vi "Grid_Main_v6.vi"(10 "Final DC":bool, 11 "Settings":T3={"Drift Correction Settings"={"Drift Correction every"=80, "Drift correction Pixels"=256, "Channel index (0-23)"=0, "MaxImagesBack"=2, "Threshold"=2, "Increment"=8, "max applied Drift Correction"=20, "Correct Drift"=TRUE, "Correlate"=0, "Correct z drift"=FALSE, "zdrift \nDuration (s)"=0.0}, "Spectroscopy Setting"={"Imaging Current"=1e-11, "ref Current"=7e-11, "tip Speed (m/s)"=2e-09, "Imaging Bias"=0.02, "ref Bias"=-0.1, "preSTS delay [ms]"=500, "STS z offset"=2e-10, "during Spec Bias (V)"=-0.1, "trigger1 < Hz"=0.0, "trigger 2 >Hz"=0.0, "autoStop"=FALSE, "Spectroscopy"=0, "PLL ON/OFF"=TRUE, "readjust setpoint every "=1, "z Reference (constHeight)"=FALSE, "Lock In"=TRUE}, "Misc"={"File name"="symmetric_node_zOff=200p", "Email when finished"="cornelius.krull@monash.edu,Dhaneesh.Gopalakrishnan@monash.edu,marina.castelli@monash.edu"}, "Grid Settings"={"type"=1, "type order"=1, "X pixel"=0, "Y pixel"=0, "Grid_Parms"={"center X (m)"=0.0, "center Y (m)"=0.0, "width (m)"=0.0, "height (m)"=0.0, "angle (deg)"=0.0}}} {"Grid Settings"."type order" items=["Grid", "Random", "Adam7"]; "Grid Settings"."type" items=["Line", "Grid", "Cloud"]; "Spectroscopy Setting"."Spectroscopy" items=["Bias", "zSpec"]; "Spectroscopy Setting"."trigger 2 >Hz" format="%#_6p"; "Spectroscopy Setting"."trigger1 < Hz" format="%#_6p"; "Spectroscopy Setting"."during Spec Bias (V)" format="%#_5p"; "Spectroscopy Setting"."STS z offset" format="%#_6p"; "Spectroscopy Setting"."ref Bias" format="%#_6p"; "Spectroscopy Setting"."Imaging Bias" format="%#_6p"; "Spectroscopy Setting"."tip Speed (m/s)" format="%.2p"; "Spectroscopy Setting"."ref Current" format="%#_6p"; "Spectroscopy Setting"."Imaging Current" format="%#_6p"; "Drift Correction Settings"."Correlate" items=["first Frame", "successive Frames"]; "Drift Correction Settings"."max applied Drift Correction" min=1 max=100 step=1 format="%.0p"; "Drift Correction Settings"."Threshold" min=1 step=1; "Drift Correction Settings"."Channel index (0-23)" items=["Current"=0, "Z (m)"=14]}) -> (3 "Settings out":T2)   [LabVIEW 2014]
uses:
  <userlib>/Nanonis Prog Interface V5/Nanonis Prog Interface.lvlib
panel:
  in  "resume":T1
  in  "stop":bool
  out "total points":i32
  out "Points taken":i32
  out "ETA":timestamp=timestamp(3575267058.899443 s since 1904-01-01)
  out "remaining time":dbl format="%<%H:%M:%S>t"
  out "Progress":u8(slide)=100 scale=0.0..100.0 scale format="%#.1g"
  out "Last z adjustment":dbl
  out "Last Drift detected (images back)":i32
  out "Y Offset out":sgl format="%#_6p"
  out "X Offset out":sgl format="%#_6p"
  out "Drift Correction Image":picture
  # "RUN smart tilt before starting the GRID\nImg Angle = 0  CHECK CUTOFF\nmove tip to reference point for tip height"
  # "%"
  # "finish the last action and then"
  # "GRID points"
  # "Increase this if no Drift was detected for \na certain number of images"
  # "% of image size"
  # "Only first frame works"
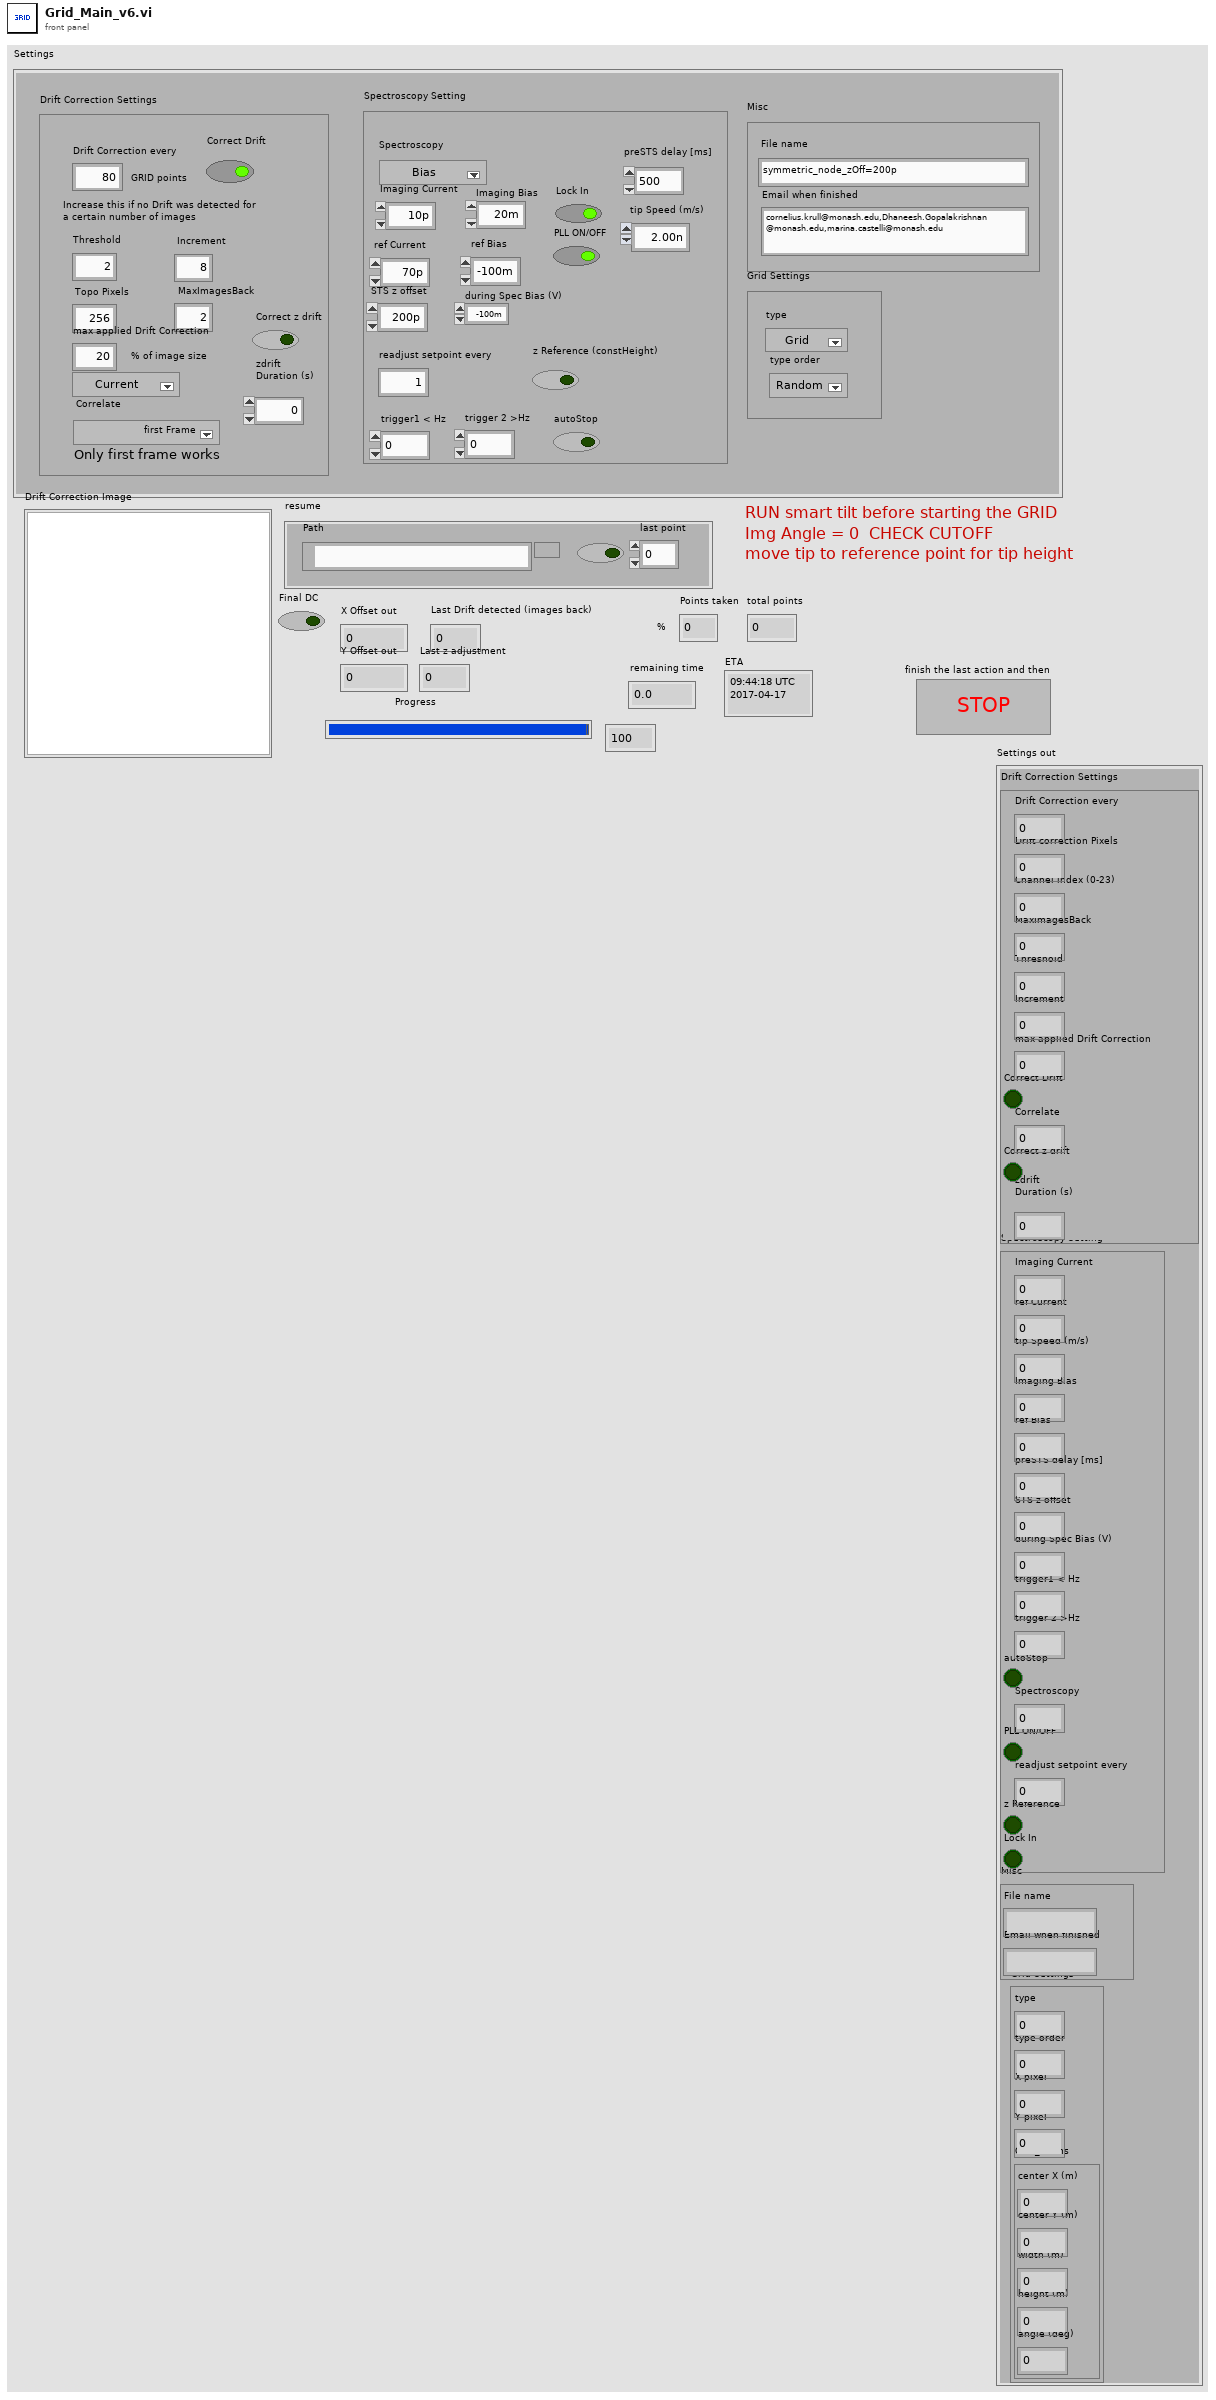
[diagram p1: front panel]
types:
  T1 = cluster{"resume Grid":bool, "Path":path, "last point":i32}
  T2 = cluster{"Drift Correction Settings":cluster{"Drift Correction every":i32, "Drift correction Pixels":i32, "Channel index (0-23)":u8, "MaxImagesBack":i32, "Threshold":i32, "Increment":i32, "max applied Drift Correction":i32, "Correct Drift":bool, "Correlate":u16, "Correct z drift":bool, "zdrift \nDuration (s)":dbl}, "Spectroscopy Setting":cluster{"Imaging Current":dbl, "ref Current":dbl, "tip Speed (m/s)":sgl, "Imaging Bias":dbl, "ref Bias":dbl, "preSTS delay [ms]":u32, "STS z offset":dbl, "during Spec Bias (V)":sgl, "trigger1 < Hz":sgl, "trigger 2 >Hz":sgl, "autoStop":bool, "Spectroscopy":u16, "PLL ON/OFF":bool, "readjust setpoint every ":i32, "z Reference":bool, "Lock In":bool}, "Misc":cluster{"File name":string, "Email when finished":string}, "Grid Settings":cluster{"type":u16, "type order":u16, "X pixel":i32, "Y pixel":i32, "Grid_Parms":cluster{"center X (m)":sgl, "center Y (m)":sgl, "width (m)":sgl, "height (m)":sgl, "angle (deg)":sgl}}}
  T3 = cluster{"Drift Correction Settings":cluster{"Drift Correction every":i32, "Drift correction Pixels":i32, "Channel index (0-23)":u8, "MaxImagesBack":i32, "Threshold":i32, "Increment":i32, "max applied Drift Correction":i32, "Correct Drift":bool, "Correlate":u16, "Correct z drift":bool, "zdrift \nDuration (s)":dbl}, "Spectroscopy Setting":cluster{"Imaging Current":dbl, "ref Current":dbl, "tip Speed (m/s)":sgl, "Imaging Bias":dbl, "ref Bias":dbl, "preSTS delay [ms]":u32, "STS z offset":dbl, "during Spec Bias (V)":sgl, "trigger1 < Hz":sgl, "trigger 2 >Hz":sgl, "autoStop":bool, "Spectroscopy":u16, "PLL ON/OFF":bool, "readjust setpoint every ":i32, "z Reference (constHeight)":bool, "Lock In":bool}, "Misc":cluster{"File name":string, "Email when finished":string}, "Grid Settings":cluster{"type":u16, "type order":u16, "X pixel":i32, "Y pixel":i32, "Grid_Parms":cluster{"center X (m)":sgl, "center Y (m)":sgl, "width (m)":sgl, "height (m)":sgl, "angle (deg)":sgl}}}
  T4 = cluster{"Drift File out":refnum<file>, "zFile":refnum<file>, "BinFile ref":refnum<file>, "xyFile":refnum<file>}
  T5 = cluster{"Drift Correction every":i32, "Drift correction Pixels":i32, "Channel index (0-23)":u8, "MaxImagesBack":i32, "Threshold":i32, "Increment":i32, "max applied Drift Correction":i32, "Correct Drift":bool, "Correlate":u16, "Correct z drift":bool, "zdrift \nDuration (s)":dbl}
  T6 = cluster{"Imaging Current":dbl, "ref Current":dbl, "tip Speed (m/s)":sgl, "Imaging Bias":dbl, "ref Bias":dbl, "preSTS delay [ms]":u32, "STS z offset":dbl, "during Spec Bias (V)":sgl, "trigger1 < Hz":sgl, "trigger 2 >Hz":sgl, "autoStop":bool, "Spectroscopy":u16, "PLL ON/OFF":bool, "readjust setpoint every ":i32, "z Reference":bool, "Lock In":bool}
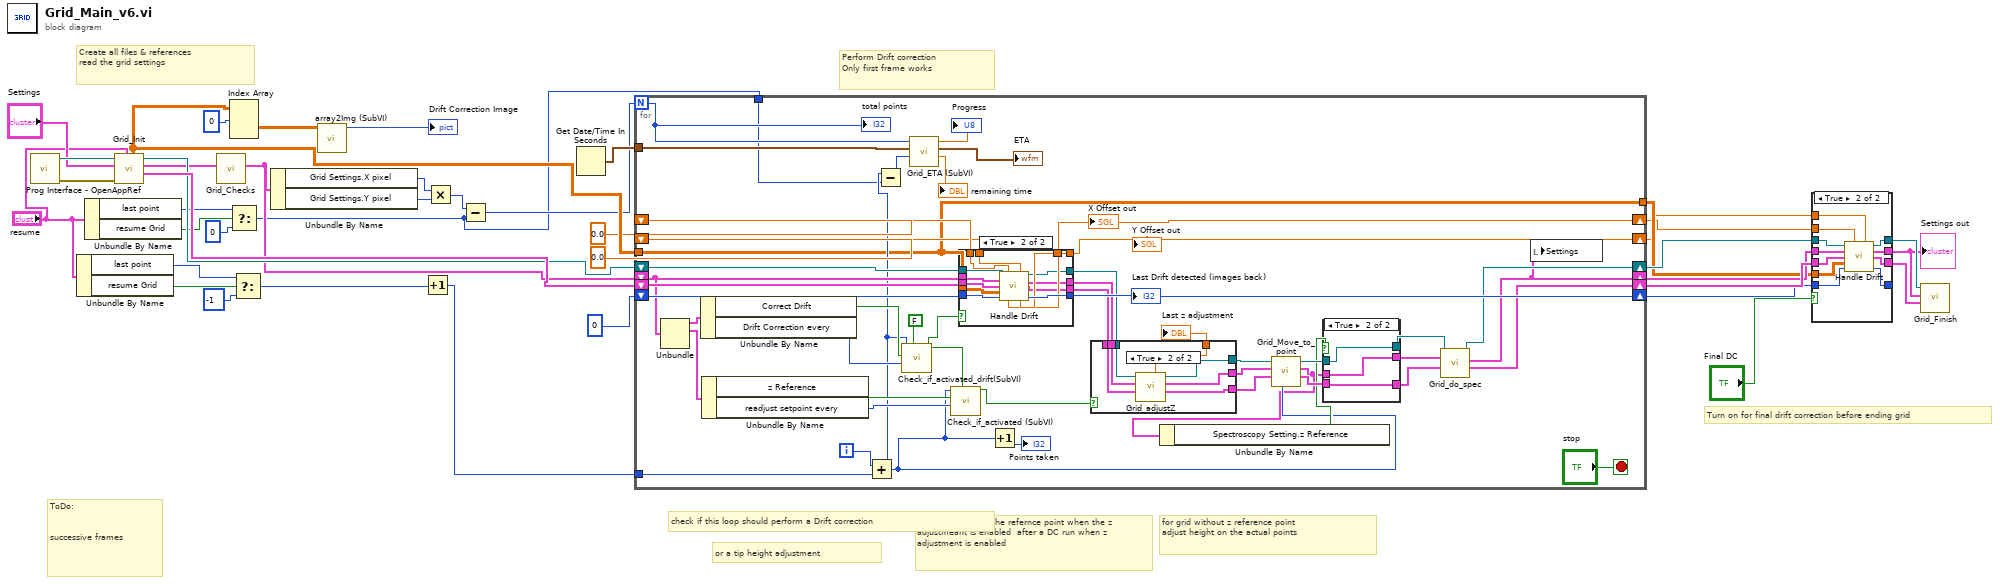
[diagram p0: block diagram]
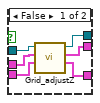
[diagram p3: hidden frame]
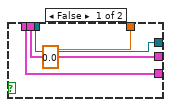
[diagram p4: hidden frame]
diagram:
  # "Turn on for final drift correction before ending grid"
  # "ToDo:\n\n\nsuccessive frames"
  # "Perform Drift correction\nOnly first frame works"
  # "check if this loop should perform a Drift correction"
  # "for grid without z reference point \nadjust height on the actual points"
  # "or a tip height adjustment"
  # "Create all files & references\nread the grid settings"
  # "adjust z height on the refernce point when the z adjustmeant is enabled  after a DC run when z adjustment is enabled"
  n1 = call <userlib>:"Prog Interface - OpenAppRef.vi"() -> ("Error out"=w39:errorcluster, "Application reference"=w40:refnum<vi>)  [unwired: 6 in]
  n2 = Unbundle By Name("resume") -> ("last point"=w21:i32, "resume Grid"=w23:bool)
  n3 = Unbundle By Name("resume") -> ("last point"=w15:i32, "resume Grid"=w17:bool)
  n4 = call "Grid_Init.vi"("resume"="resume", "Error in"=w39, "Settings"="Settings", "Application reference"=w40) -> ("FileRefs"=w37:T4, "Settings out"=w26:T2, "Application ref out"=w36:refnum<vi>, "DC images"=w34:dbl[][][])  [unwired: 3 in, 1 out]
  n5 = call "Grid_Checks.vi"("Settings"=w26) -> ("Settings out"=w25:T2)  [unwired: 10 in]
  n6 = Index Array(array=w34, index (dim 0)=0 ("index (page)")) -> (element=w35:dbl[][])  [unwired: 2 in]
  n7 = Select(t=w15, s=w17, f=0) -> (s? t:f=w12:i32)
  n8 = Select(t=w21, s=w23, f=-1) -> (s? t:f=w20:i32)
  n9 = Unbundle By Name(w25) -> ("Grid Settings.X pixel"=w29:i32, "Grid Settings.Y pixel"=w28:i32)
  n10 = call "array2Img (SubVI).vi"("Rxy"=w35) -> ("new picture"=→"Drift Correction Image":picture)  [unwired: 10 in]
  n11 = Increment(x=w20) -> (x+1=w18:i32)
  n12 = Multiply(x=w29, y=w28) -> (x*y=w13:i32)
  n13 = Subtract(x=w13, y=w12) -> (x-y=w19:i32)
  n14 = Get Date/Time In Seconds() -> (seconds since 1Jan1904=w27:timestamp)
  n15 = for {
    N: w19 -> [w47]
    tunnel: w34 -> [w41]
    shift-right: [w86] -> w7
    shift-left: 0 ("Last Drift out") -> [w85]
    shift-right: [w81] -> w5
    shift-left: sgl 0.0 ("X Offset out") -> [w84]
    shift-right: [w82] -> w4
    shift-left: sgl 0.0 ("Y Offset out") -> [w83]
    tunnel: w27 -> [w72]
    shift-right: [w69] -> w9
    shift-left: w36 -> [w87]
    shift-right: [w43] -> w10
    shift-left: w25 -> [w54]
    shift-right: [w68] -> w11
    shift-left: w37 -> [w88]
    tunnel: w18 -> [w55]
    tunnel: w12 -> [w44]
    tunnel: [w41] -> w6
    i -> [w66]
    stop <- "stop" stop-if-true
    n16 = Unbundle(w54) -> ("Drift Correction Settings"=w53:T5, "Spectroscopy Setting"=w51:T6)  [unwired: 2 out]
    n17 = Unbundle By Name(w53) -> ("Correct Drift"=w52:bool, "Drift Correction every"=w48:i32)
    n18 = Unbundle By Name(w51) -> ("z Reference"=w50:bool, "readjust setpoint every"=w49:i32)
    n19 = Add(x=w66, y=w55) -> (x+y=w45:i32)
    n20 = Subtract(x=w45, y=w44) -> (x-y=w46:i32)
    n21 = call "Check_if_activated_drift(SubVI).vi"("Override"=FALSE, "activate  every  iterations"=w48, "activated?"=w52, "Iteration"=w45) -> ("perform action"=w77:bool)  [unwired: 7 in]
    n22 = call "Grid_ETA (SubVI).vi"("points taken"=w46, "seconds since 1Jan1904"=w72, "points todo"=w47) -> ("Numeric 4"=→"remaining time":dbl, "Time Stamp"=→"ETA":timestamp, "Numeric 3"=→"Progress":dbl)  [unwired: 6 in]
    n23 = call "Check_if_activated (SubVI).vi"("Override"=w77, "activate  every  iterations"=w49, "activated?"=w50, "Iteration"=w45) -> ("perform action"=w78:bool)  [unwired: 7 in]
    n24 = case shown="True" w77 {
      tunnel: w54 -> [w111 w127]
      tunnel: w88 -> [w110 w126]
      tunnel: w87 -> [w109 w125]
      tunnel: w41 -> [_ w124]
      tunnel: [w112 w123] -> w86
      tunnel: w85 -> [w112 w122]
      tunnel: w84 -> [w114 w121]
      tunnel: w83 -> [w113 w120]
      tunnel: [w113 w119] -> w82
      tunnel: [w114 w118] -> w81
      tunnel: [w109 w117] -> w80
      tunnel: [w111 w116] -> w57
      tunnel: [w110 w115] -> w79
      frame False {
      }
      frame True {
        n25 = call "Handle Drift.vi"("Application ref in"=w125, "X Offset in"=w121, "Y Offset In"=w120, "Settings"=w127, "FileRefs"=w126, "Drift Correction image"=w124, "Last Drift"=w122) -> ("Application out"=w117:refnum<vi>, "Settings out"=w116:T2, "FileRefs out File Refs  Out"=w115:T4, "X Offset out"=w118:sgl, "Y Offset out"=w119:sgl, "Last Drift out"=w123:i32)  [unwired: 3 in]
      }
    }
    "X Offset out" <- w81
    "Y Offset out" <- w82
    "Last Drift detected (images back)" <- w86
    n26 = Increment(x=w45) -> (x+1=→"Points taken":i32)
    n27 = case shown="True" w78 {
      tunnel: w80 -> [w100 w108]
      tunnel: w79 -> [w99 w107]
      tunnel: w57 -> [w98 w106]
      tunnel: [w99 w105] -> w71
      tunnel: [w98 w104] -> w59
      tunnel: [w100 w103] -> w70
      tunnel: [0.0 ("Last z adjustment") w102] -> w67
      frame False {
      }
      frame True {
        n28 = call "Grid_adjustZ.vi"("FileRefs"=w107, "Settings"=w106, "Application in"=w108) -> ("FileRefs out"=w105:T4, "Settings out"=w104:T2, "Application ref out"=w103:refnum<vi>, "Last z adjustment"=w102:dbl)  [unwired: 4 in, 1 out]
      }
    }
    "Last z adjustment" <- w67
    n29 = call "Grid_Move_to_point.vi"("point"=w45, "FileRefs in"=w71, "Settings"=w59, "Application ref in"=w70) -> ("FileRefs out"=w61:T4, "Settings out"=w42:T2, "Application ref out"=w62:refnum<vi>)  [unwired: 5 in]
    n30 = Unbundle By Name(w42) -> ("Spectroscopy Setting.z Reference"=w60:bool)
    n31 = case shown="True" w60 {
      tunnel: [w94 w97] -> w65
      tunnel: [w93 w95] -> w63
      tunnel: [w92 w96] -> w64
      tunnel: w62 -> [w91 w97]
      tunnel: w42 -> [w90 w96]
      tunnel: w61 -> [w89 w95]
      frame False {
        n32 = call "Grid_adjustZ.vi"("FileRefs"=w89, "Settings"=w90, "Application in"=w91) -> ("FileRefs out"=w93:T4, "Settings out"=w92:T2, "Application ref out"=w94:refnum<vi>)  [unwired: 4 in, 2 out]
      }
      frame True {
      }
    }
    n33 = call "Grid_do_spec.vi"("FileRefs in"=w63, "Settings in"=w64, "Application ref in"=w65) -> ("FileRefs out"=w68:T4, "Settings out"=w43:T2, "Application ref out"=w69:refnum<vi>)  [unwired: 5 in, 1 out]
    n34 = local write "Settings"(w43) -> ()
    "total points" <- w47
  }
  n35 = case shown="True" "Final DC" {
    tunnel: w10 -> [w130 w142]
    tunnel: w11 -> [w129 w141]
    tunnel: w9 -> [w128 w140]
    tunnel: [w131 w139] -> _
    tunnel: w7 -> [w131 w135]
    tunnel: [w128 w138] -> w8
    tunnel: [w130 w137] -> w2
    tunnel: [w129 w136] -> w3
    tunnel: w6 -> [_ w134]
    tunnel: w5 -> [_ w133]
    tunnel: w4 -> [_ w132]
    frame False {
    }
    frame True {
      n36 = call "Handle Drift.vi"("Application ref in"=w140, "X Offset in"=w133, "Y Offset In"=w132, "Settings"=w142, "FileRefs"=w141, "Drift Correction image"=w134, "Last Drift"=w135) -> ("Application out"=w138:refnum<vi>, "Settings out"=w137:T2, "FileRefs out File Refs  Out"=w136:T4, "Last Drift out"=w139:i32)  [unwired: 3 in, 2 out]
    }
  }
  "Settings out" <- w2
  n37 = call "Grid_Finish.vi"("FileRefs"=w3, "Settings"=w2, "Application reference"=w8) -> ()  [unwired: 9 in]
